vi "Handle Serial Errors.vi"(7 "GV State":enum16{"Init", "Test"}(ring)=enum."Test", 8 "error in":errorcluster, 10 "Ctl Refs":T1, 11 "Port":refnum<visa-resource-name>) -> (0 "Error Out":errorcluster, 1 "Version":string, 2 "Reconnect?":bool, 3 "Port 2":refnum<visa-resource-name>)   [LabVIEW 2013]
doc: "This VI is a functional global that handles disconects on the serial line. If there is a disconnect, then the system will send commands to return to the previous altitude and mode upon reconnection. \n\nThe FGV takes references to three input controls: the altitude setpoint, mode and the confirmation of altitude change buttons. When an error is thrown upon a serial communication attempt, the current values of the controls will be stored and a flag is raised. When communication is restored, the FGV will send commands to the controls in this order: altitude, confirmation, and mode. Once this is complete, it will clear the raised flag.\n\nTwo types of errors are raised - one is when something happens to the connection on the serial side, i.e. the CAT engine becomes disconnected from the computer at the serial port on the engine. The other occurs when the USB becomes disconnected (error -1073807194). This one requires a closing of the initial connection to the port and then attempting to reconnect based on a query of available connections.\n\nIn the latter case, the"
uses:
  MSR/VertMode/VertMode.xctl
  Type Defs/Alt Control.ctl
  Type Defs/Alt Digit 100 New.ctl
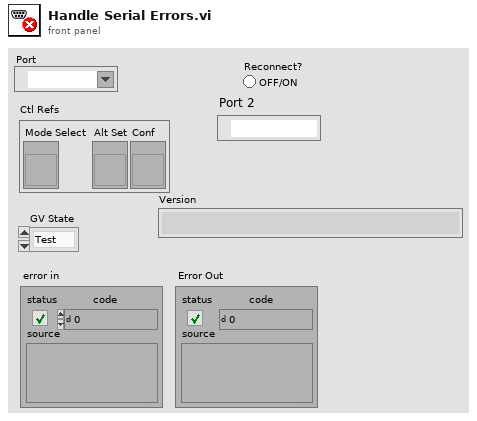
[diagram p1: front panel]
types:
  T1 = cluster{"Mode Select":refnum<vi>, "Alt Set":refnum<vi>, "Conf":refnum<vi>}
  T2 = typedef "Alt Control.ctl" = cluster{"Alt Digit 100":T3, "Alt Digit 100":T3, "Alt Digit 100":T3, "Alt Digit 100":T3, "Alt Digit 100":T3}
  T3 = typedef "Alt Digit 100 New.ctl" = i8
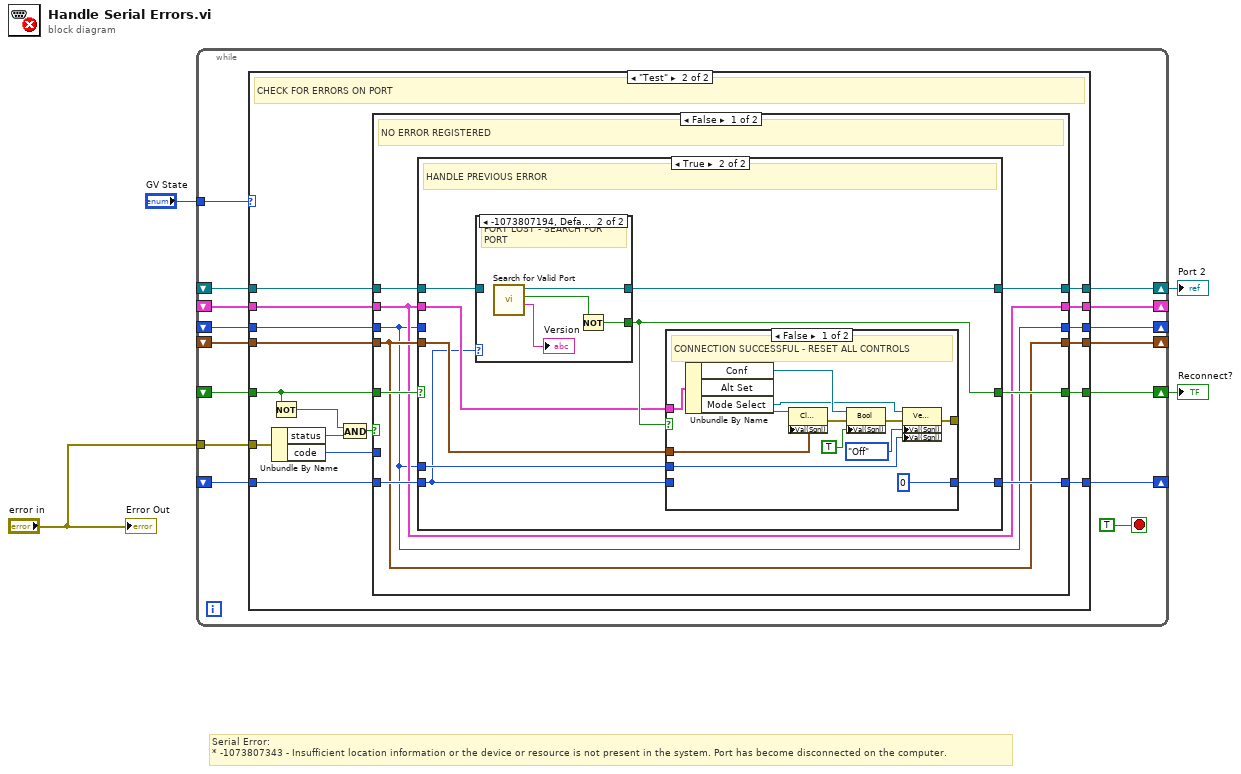
[diagram p0: block diagram]
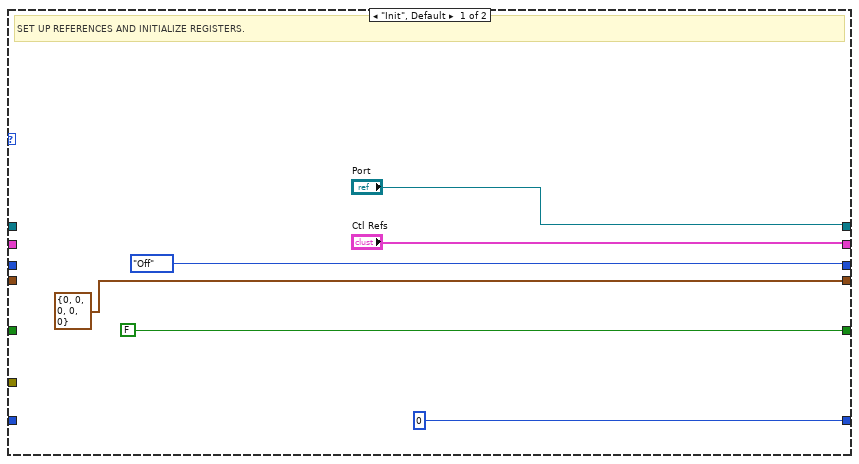
[diagram p2: hidden frame]
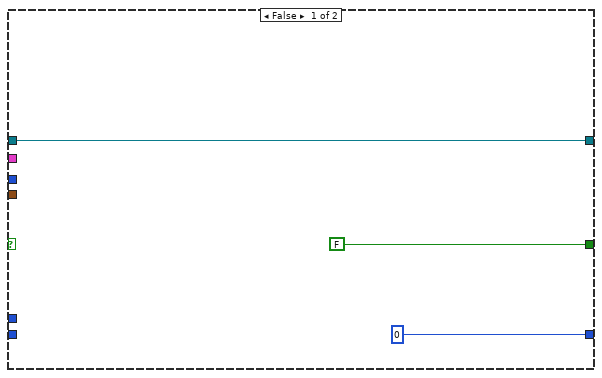
[diagram p3: hidden frame]
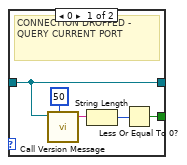
[diagram p5: hidden frame]
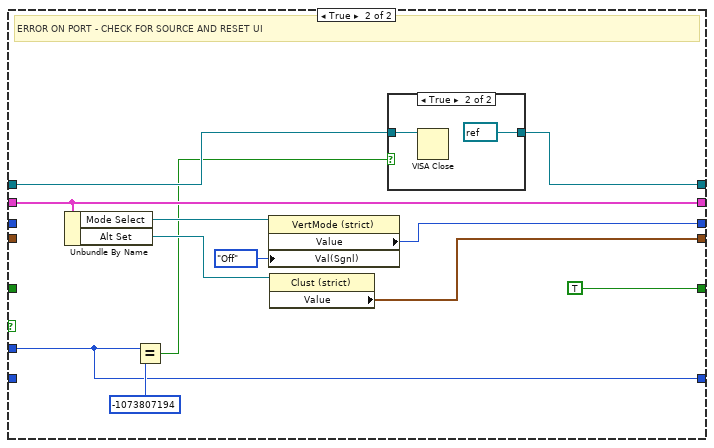
[diagram p6: hidden frame]
diagram:
  # "Serial Error:\n* -1073807343 - Insufficient location information or the device or resource is not present in the system. Port has become disconnected on the computer."
  n1 = while {
    tunnel: "error in" -> [w19]
    shift-right: [w18] -> w2
    shift-left: _ -> [w13]
    tunnel: "GV State" -> [w17]
    shift-right: [w16] -> _
    shift-left: _ -> [w15]
    shift-right: [w14] -> _
    shift-left: _ -> [w10]
    shift-right: [w12] -> _
    shift-left: _ -> [w9]
    shift-right: [w8] -> w1
    shift-left: _ -> [w7]
    shift-right: [w6] -> _
    shift-left: _ -> [w5]
    stop <- TRUE stop-if-true
    n2 = case shown="\"Test\"" w17 {
      tunnel: w19 -> [_ w31]
      tunnel: [FALSE w42] -> w18
      tunnel: ["Ctl Refs" w36] -> w16
      tunnel: w15 -> [_ w41]
      tunnel: [enum8{"Off", "Stby", "Hold", "Run"}."Off" ("Value") w40] -> w14
      tunnel: w13 -> [_ w32]
      tunnel: [T2 {"Alt Digit 100"=0, "Alt Digit 100"=0, "Alt Digit 100"=0, "Alt Digit 100"=0, "Alt Digit 100"=0} ("Value") w39] -> w12
      tunnel: w10 -> [_ w38]
      tunnel: w9 -> [_ w37]
      tunnel: ["Port" w34] -> w8
      tunnel: w7 -> [_ w35]
      tunnel: [0 ("code") w27] -> w6
      tunnel: w5 -> [_ w26]
      frame "Init", Default {
        # "SET UP REFERENCES AND INITIALIZE REGISTERS."
      }
      frame "Test" {
        # "CHECK FOR ERRORS ON PORT"
        n3 = Not(x=w32) -> (.not. x?=w33:bool)
        n4 = Unbundle By Name(w31) -> ("status"=w30:bool, "code"=w28:i32)
        n5 = And(x=w33, y=w30) -> (x .and. y?=w29:bool)
        n6 = case shown="False" w29 {
          tunnel: [w49 TRUE] -> w42
          tunnel: w41 -> [w44 w91]
          tunnel: [w43 w93] -> w40
          tunnel: w32 -> [w51 _]
          tunnel: [w45 w92] -> w39
          tunnel: w38 -> [w43 _]
          tunnel: w37 -> [w45 _]
          tunnel: [w44 w91] -> w36
          tunnel: w35 -> [w50 w88]
          tunnel: [w48 w87] -> w34
          tunnel: w28 -> [_ w85]
          tunnel: [w46 w85] -> w27
          tunnel: w26 -> [w47 _]
          frame False {
            # "NO ERROR REGISTERED"
            n7 = case shown="True" w51 {
              tunnel: w44 -> [_ w59]
              tunnel: w43 -> [_ _]
              tunnel: w45 -> [_ w57]
              tunnel: w50 -> [w54 w62]
              tunnel: [FALSE w60] -> w49
              tunnel: [w54 w61] -> w48
              tunnel: w47 -> [_ w55]
              tunnel: [0 ("code") w56] -> w46
              tunnel: w43 -> [_ w58]
              frame False {
              }
              frame True {
                # "HANDLE PREVIOUS ERROR"
                n8 = case shown="-1073807194, Default" w55 {
                  tunnel: w62 -> [w77 _]
                  tunnel: [w76 w84] -> w60
                  tunnel: [w77 w83] -> w61
                  frame 0 {
                    # "CONNECTION DROPPED - QUERY CURRENT PORT"
                    n9 = call "Call Version Message.vi"("VISA resource name out"=w77, "delay before read (ms)"=u32 50) -> ("read string"=w79:string)  [unwired: 3 in, 3 out]
                    n10 = String Length(string=w79) -> (length=w78:i32)
                    n11 = Less Or Equal To 0?(x=w78) -> (x <= 0?=w76:bool)
                  }
                  frame -1073807194, Default {
                    # "PORT LOST - SEARCH FOR PORT"
                    n12 = call "Search for Valid Port.vi"() -> ("Version"=→"Version":string, "CAT Port?"=w82:bool, "Port Out"=w83:refnum<visa-resource-name>)  [unwired: 9 in]
                    n13 = Not(x=w82) -> (.not. x?=w84:bool)
                  }
                }
                n14 = case shown="False" w60 {
                  tunnel: w59 -> [w74 _]
                  tunnel: w57 -> [w69 _]
                  tunnel: w58 -> [w65 _]
                  tunnel: w55 -> [_ w75]
                  tunnel: [0 ("code") w75] -> w56
                  tunnel: [w63 _] -> _
                  frame False {
                    # "CONNECTION SUCCESSFUL - RESET ALL CONTROLS"
                    n15 = Unbundle By Name(w74) -> ("Conf"=w72:refnum<vi>, "Alt Set"=w73:refnum<vi>, "Mode Select"=w67:refnum<vi>)
                    n16 = property class="Clust (strict)"(reference=w73, "Val(Sgnl)"=w69) -> (error out=w71:errorcluster)  [unwired: 1 in, 1 out]
                    n17 = property class="Bool"(reference=w72, error in=w71, "Val(Sgnl)"=TRUE ("Value (Signaling)")) -> (error out=w68:errorcluster)  [unwired: 1 out]
                    n18 = property class="VertMode (strict)"(reference=w67, error in=w68, "Val(Sgnl)"=enum8{"Off", "Stby", "Hold", "Run"}."Off" ("Value (Signaling)"), "Val(Sgnl)"=w65) -> (error out=w63:errorcluster)  [unwired: 1 out]
                  }
                  frame True {
                    # "INVALID RESPONSE TO VERSION REQUEST"
                  }
                }
              }
            }
          }
          frame True {
            # "ERROR ON PORT - CHECK FOR SOURCE AND RESET UI"
            n19 = Unbundle By Name(w91) -> ("Mode Select"=w95:refnum<vi>, "Alt Set"=w94:refnum<vi>)
            n20 = Equal?(x=w85, y=-1073807194 ("x")) -> (x = y?=w86:bool)
            n21 = property class="VertMode (strict)"(reference=w95, "Val(Sgnl)"=enum8{"Off", "Stby", "Hold", "Run"}."Off" ("Value")) -> ("Value"=w93:enum8{"Off", "Stby", "Hold", "Run"})  [unwired: 1 in, 2 out]
            n22 = property class="Clust (strict)"(reference=w94) -> ("Value"=w92:T2)  [unwired: 1 in, 2 out]
            n23 = case shown="True" w86 {
              tunnel: w88 -> [w97 w99]
              tunnel: [w97 refnum<visa-resource-name> refnum ("Port")] -> w87
              frame False {
              }
              frame True {
                n24 = VISA Close(VISA resource name=w99) -> ()  [unwired: 1 in, 1 out]
              }
            }
          }
        }
      }
    }
  }
  "Reconnect?" <- w2
  "Port 2" <- w1
  "Error Out" <- "error in"
